vi "3.11-Get Max Turn Center.vi"(1 "X (mm)":dbl, 2 "Distance Along Y where polar system is centered":i32=590, 3 "Y (mm)":dbl) -> (0 "Start Turn Angle":dbl)   [LabVIEW 2010]
uses:
  3.0-Global.vi
panel:
  out "Center of Max Turn arc":dbl
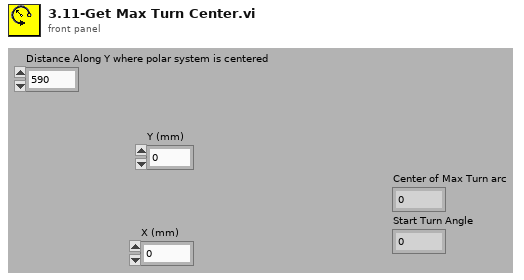
[diagram p1: front panel]
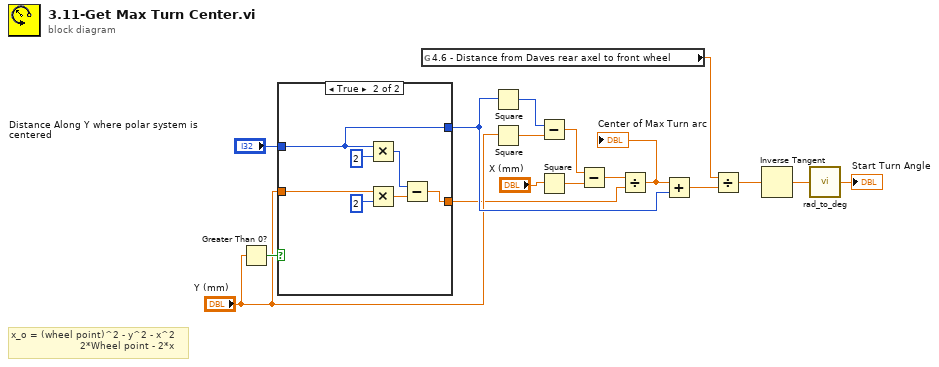
[diagram p0: block diagram]
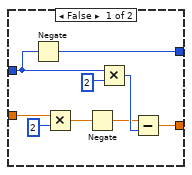
[diagram p2: hidden frame]
diagram:
  # "x_o = (wheel point)^2 - y^2 - x^2\n                       2*Wheel point - 2*x"
  n1 = Greater Than 0?(x="Y (mm)") -> (x > 0?=w8:bool)
  n2 = case shown="True" w8 {
    tunnel: [w22 w28] -> w6
    tunnel: "Distance Along Y where polar system is centered" -> [w18 w28]
    tunnel: "Y (mm)" -> [w21 w29]
    tunnel: [w20 w27] -> w2
    frame False {
      n3 = Negate(x=w18) -> (-x=w22:i32)
      n4 = Multiply(x=w21, y=2) -> (x*y=w23:dbl)
      n5 = Negate(x=w23) -> (-x=w19:dbl)
      n6 = Multiply(x=w18, y=2) -> (x*y=w24:i32)
      n7 = Subtract(x=w19, y=w24) -> (x-y=w20:dbl)
    }
    frame True {
      n8 = Multiply(x=w28, y=2) -> (x*y=w30:i32)
      n9 = Multiply(x=w29, y=2) -> (x*y=w31:dbl)
      n10 = Subtract(x=w30, y=w31) -> (x-y=w27:dbl)
    }
  }
  n11 = global read "3.0-Global.vi" "4.6 - Distance from Daves rear axel to front wheel"() -> (w1:dbl)
  n12 = Square(x=w6) -> (x^2=w15:i32)
  n13 = Square(x="Y (mm)") -> (x^2=w16:dbl)
  n14 = Subtract(x=w15, y=w16) -> (x-y=w13:dbl)
  n15 = Square(x="X (mm)") -> (x^2=w14:dbl)
  n16 = Subtract(x=w13, y=w14) -> (x-y=w12:dbl)
  n17 = Divide(x=w12, y=w2) -> (x/y=w7:dbl)
  "Center of Max Turn arc" <- w7
  n18 = Add(x=w7, y=w6) -> (x+y=w5:dbl)
  n19 = Divide(x=w1, y=w5) -> (x/y=w11:dbl)
  n20 = Inverse Tangent(1:w11) -> (0:w10:dbl)
  n21 = call "rad_to_deg.vi"("Radians"=w10) -> ("Degrees"=→"Start Turn Angle":dbl)
